vi "motion_command.vi"() -> ()   [LabVIEW 2017]
panel:
  out "PlannerPath Heading":dbl
  out "Waypoint Heading":dbl
  out "Vehicle Heading":dbl
  out "Steering Ratio clac":dbl
  out "Lateral Offset Origin":dbl
  out "Inclination":dbl
  out "Distance":dbl
  out "Goal speed":dbl
  out "Speed Command":dbl
  out "Angle Difference":dbl
  out "Curvature":dbl
  out "Heading Angle":dbl
  out "Tangential Angle":dbl
  out "Lateral Offset":dbl
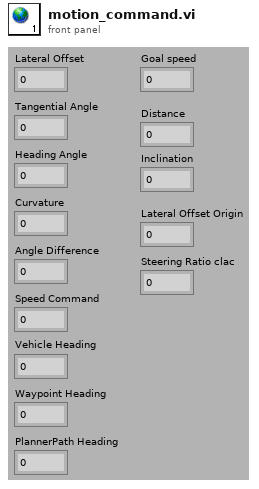
[diagram p1: front panel]
diagram:
